vi "patientListView.vi"() -> ()   [LabVIEW 2019]
uses:
  03_Home/controller/logoutBtn.ctl
  03_Home/controller/exitBtn.ctl
  <vilib>/Utility/miscctls.llb/LVPointTypeDef.ctl
  subVI/patients_state.ctl
  03_Home/controller/pannelState.ctl
  globalValue.vi
panel:
  in  "btnGroup":T1
  in  "trashBtn":bool
  in  "createBtn":bool
  in  "backPage":bool
  out "x-y*floor(x/y)":i32
  out "totalCount":string
  out "totalPage":i8
  out "crrentPage":i8
  in  "leftBtn":bool
  in  "rightBtn":bool
  out "patientList":i32(listbox)
  in  "searchBtn":bool
  in  "searchForm":string
  in  "Help Button":bool
  in  "LogOut Button":T2
  in  "Exit Button":T3
  out "userNm":string
  # "/"
  # "|"
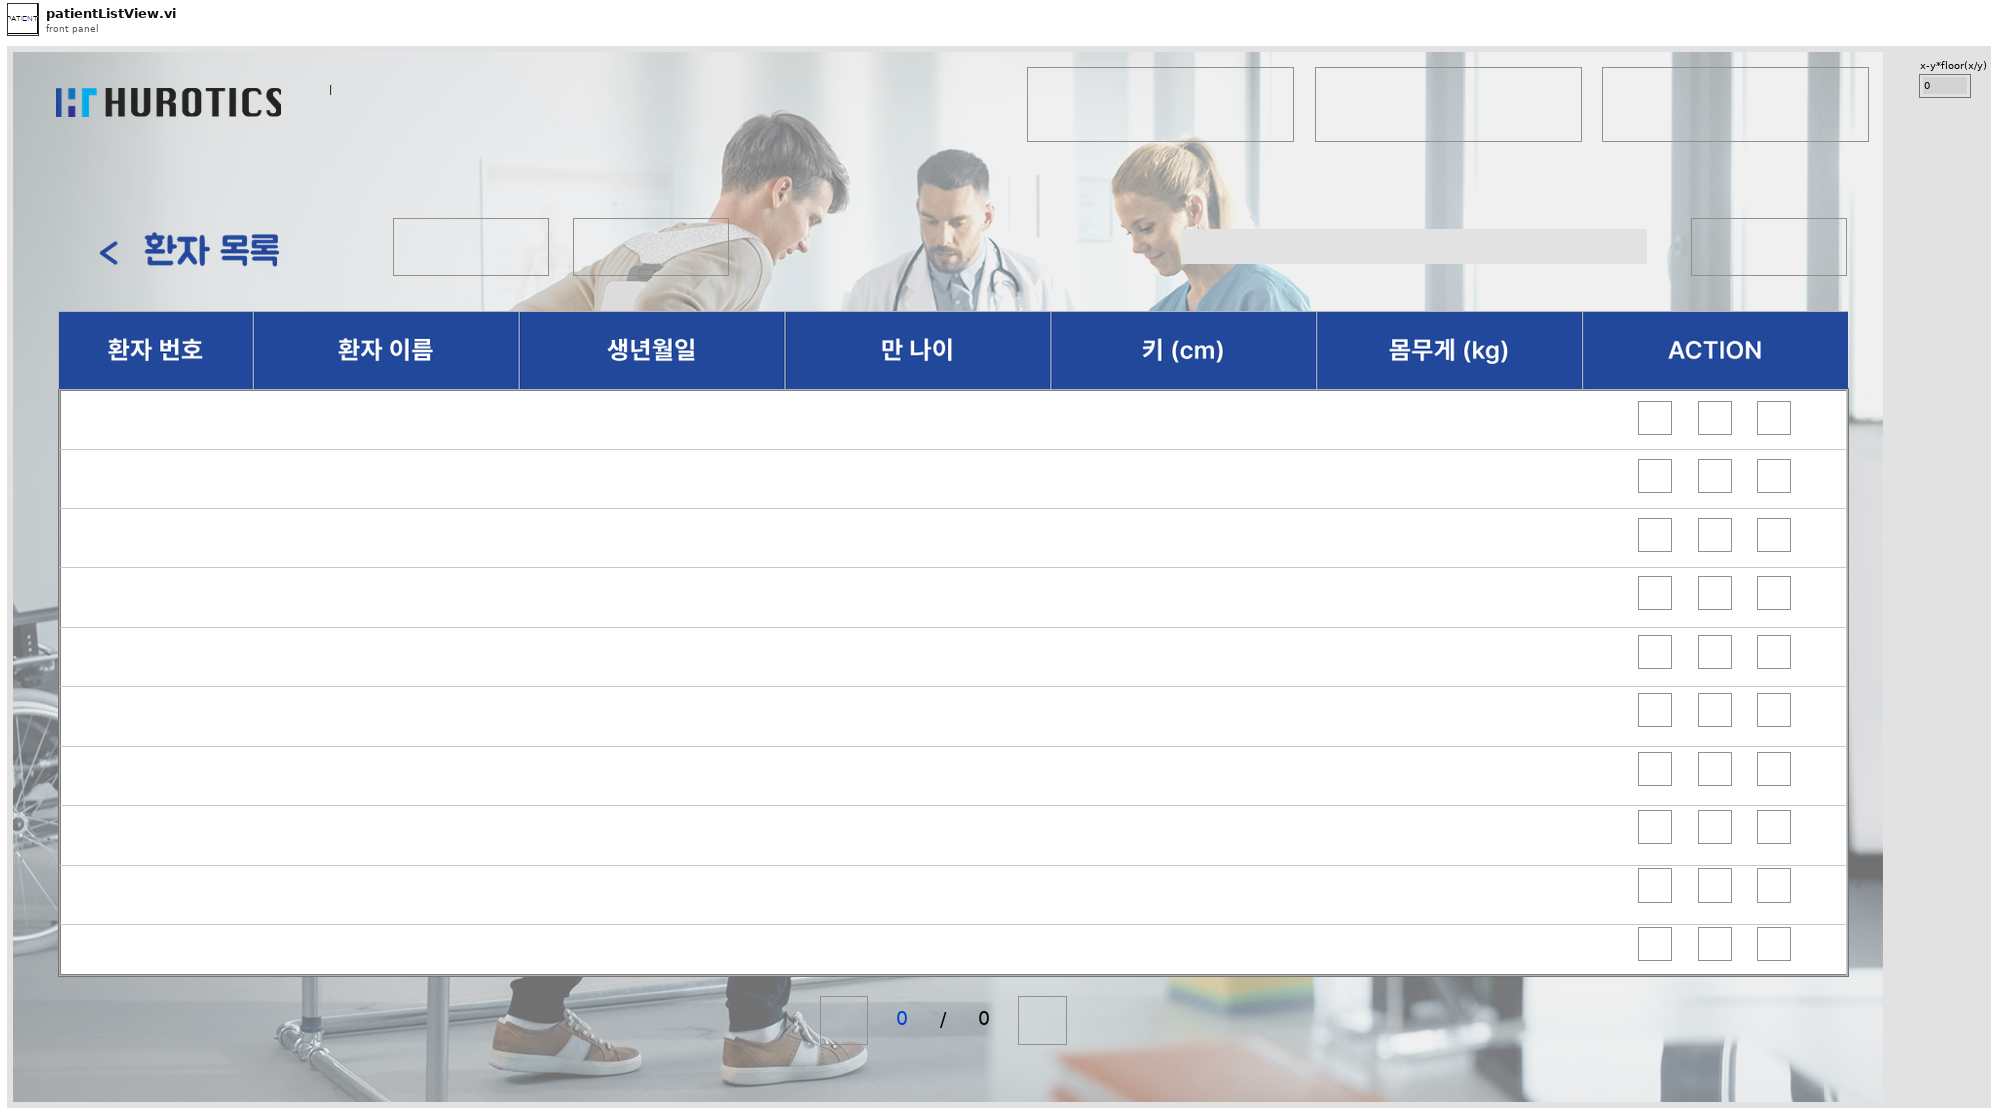
[diagram p1: front panel]
types:
  T1 = cluster{"detailBtn":bool, "updateBtn":bool, "deleteBtn":bool, "detailBtn 2":bool, "updateBtn 2":bool, "deleteBtn 2":bool, "detailBtn 3":bool, "updateBtn 3":bool, "deleteBtn 3":bool, "detailBtn 4":bool, "updateBtn 4":bool, "deleteBtn 4":bool, "detailBtn 5":bool, "updateBtn 5":bool, "deleteBtn 5":bool, "detailBtn 6":bool, "updateBtn 6":bool, "deleteBtn 6":bool, "detailBtn 7":bool, "updateBtn 7":bool, "deleteBtn 7":bool, "detailBtn 8":bool, "updateBtn 8":bool, "deleteBtn 8":bool, "detailBtn 9":bool, "updateBtn 9":bool, "deleteBtn 9":bool, "detailBtn 10":bool, "updateBtn 10":bool, "deleteBtn 10":bool}
  T2 = typedef "logoutBtn.ctl" = bool
  T3 = typedef "exitBtn.ctl" = bool
  T4 = typedef "LVPointTypeDef.ctl" = cluster{"Horizontal":i16, "Vertical":i16}
  T5 = enum16{"connection", "create", "getReadList", "getRead", "getCount", "update", "delete", "close"}
  T6 = typedef "patients_state.ctl" = enum16{"connection", "create", "getReadList", "getRead", "getCount", "update", "delete", "trash", "restore", "close"}
  T7 = enum8{"Enabled", "Disabled", "Disabled and Grayed Out"}
  T8 = typedef "pannelState.ctl" = enum16{"Init", "LogIn", "SignUpView", "Home", "Management_patientList", "Management_patientTrashtList", "Management_patientCreate", "Management_patientUpdate", "Management_patientTraining", "Management_patientTrainingDetail", "H-MEDI PatientList", "H-MEDI HardwareCtl", "Adjust", "FineTuning", "UserList", "UserDetail", "Exit"}
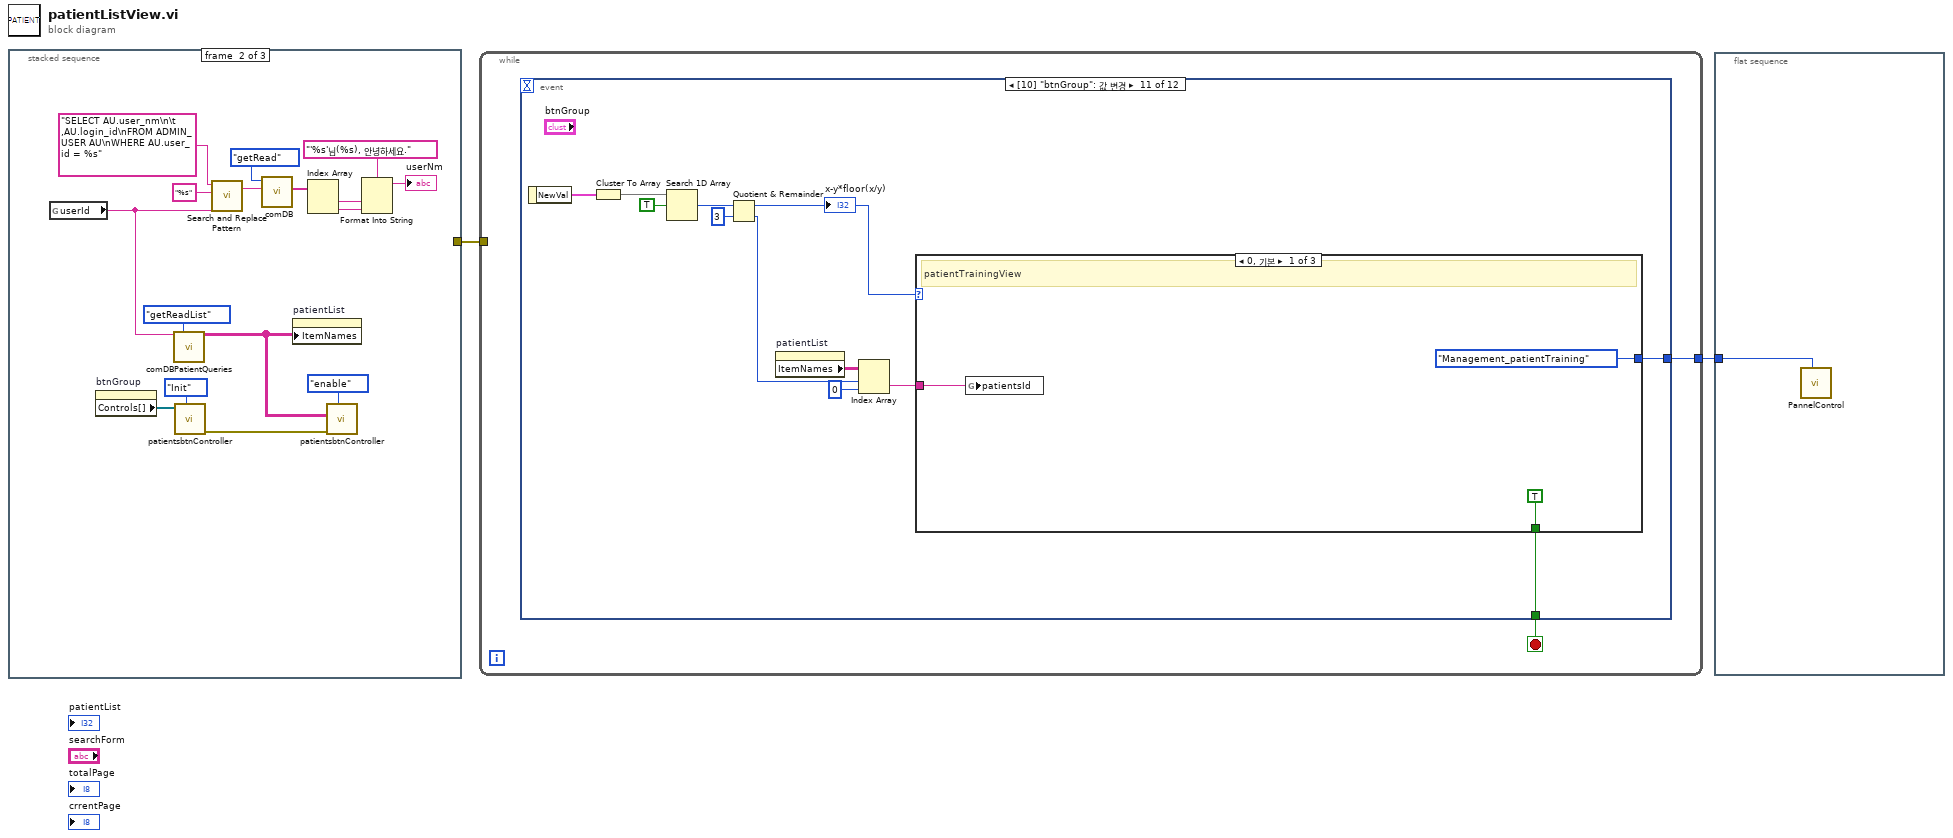
[diagram p0: block diagram]
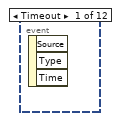
[diagram p2: hidden frame]
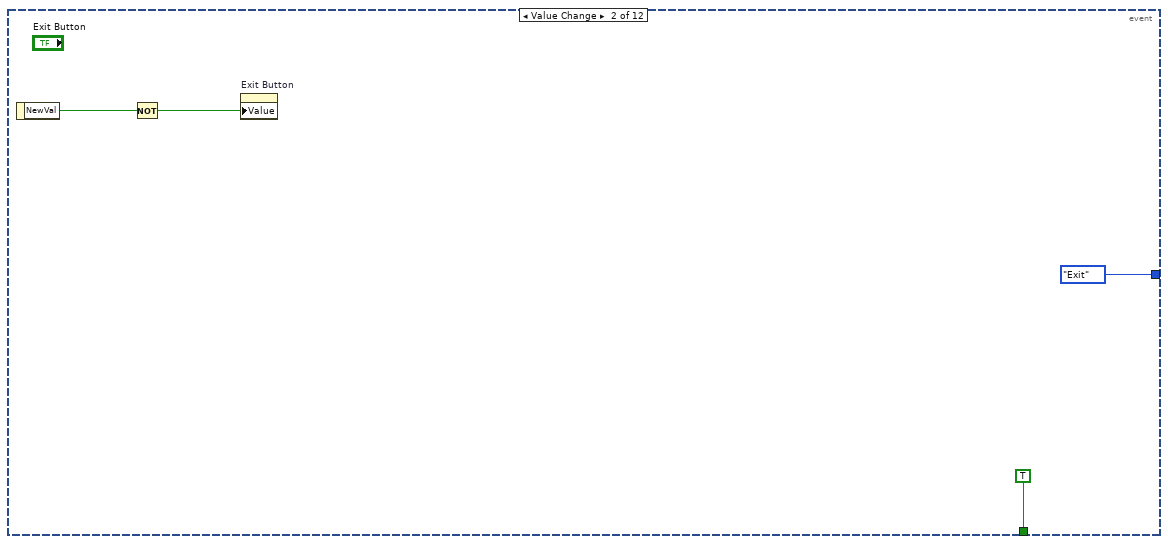
[diagram p3: hidden frame]
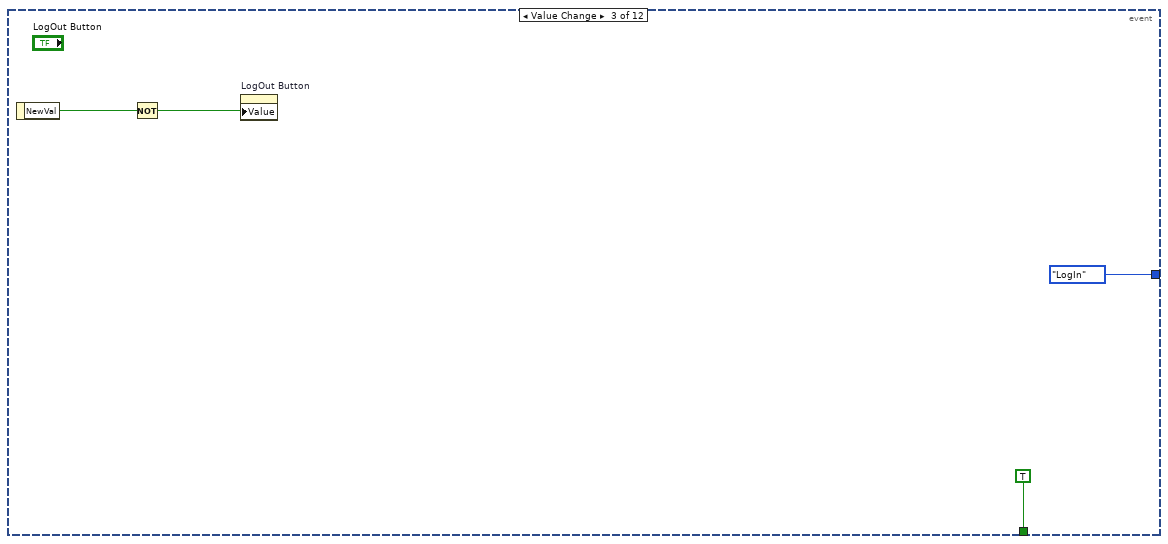
[diagram p4: hidden frame]
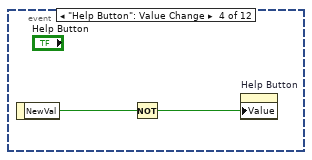
[diagram p5: hidden frame]
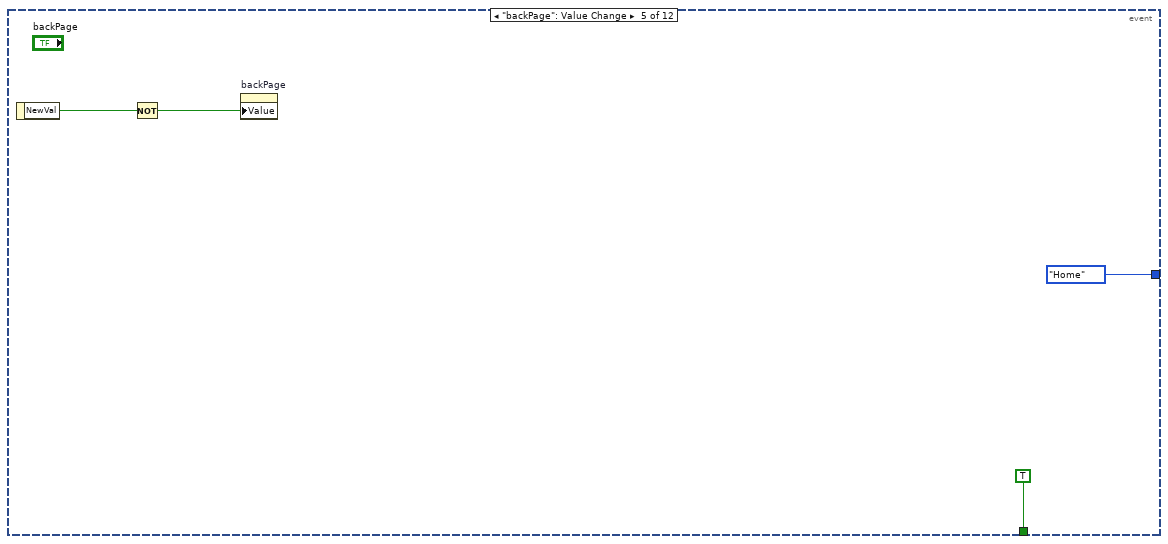
[diagram p6: hidden frame]
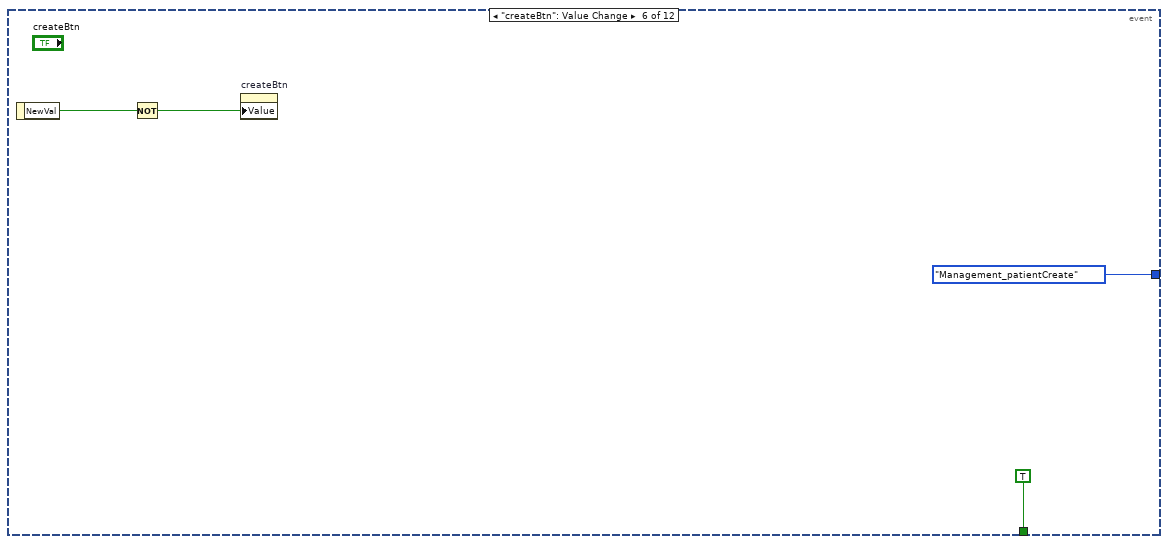
[diagram p7: hidden frame]
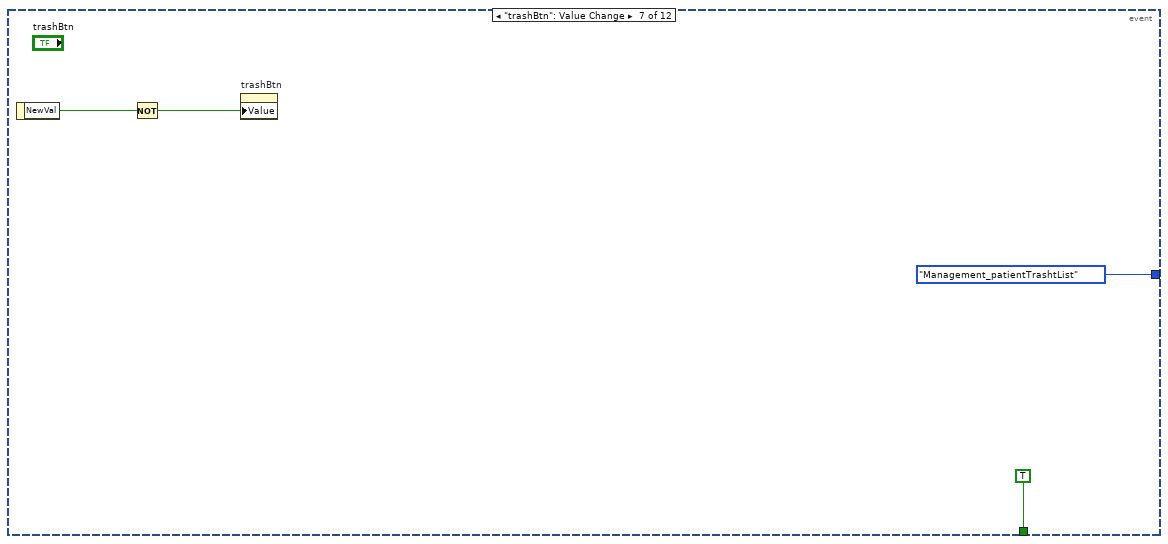
[diagram p8: hidden frame]
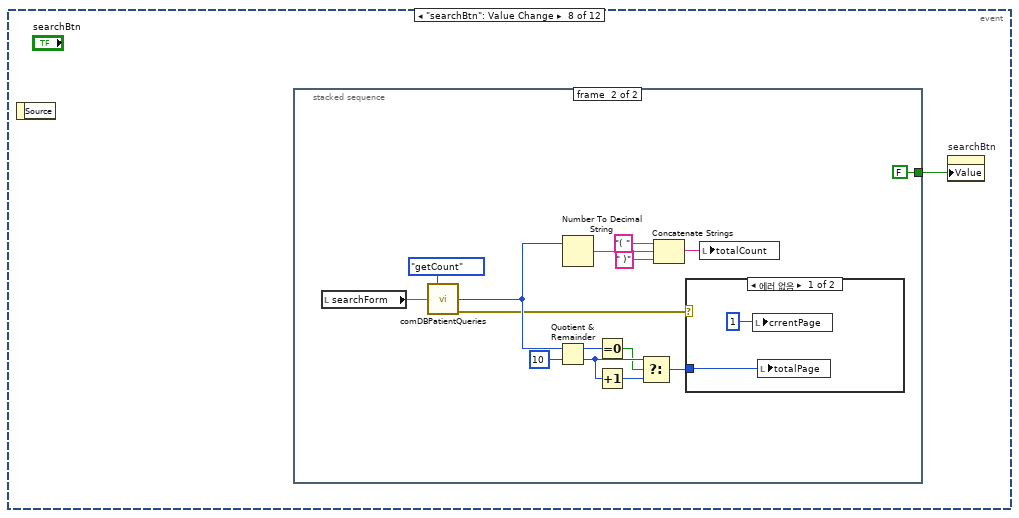
[diagram p9: hidden frame]
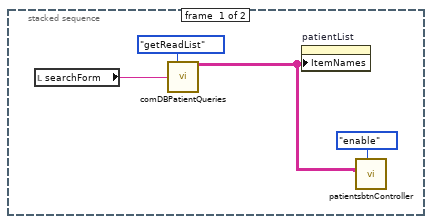
[diagram p10: hidden frame]
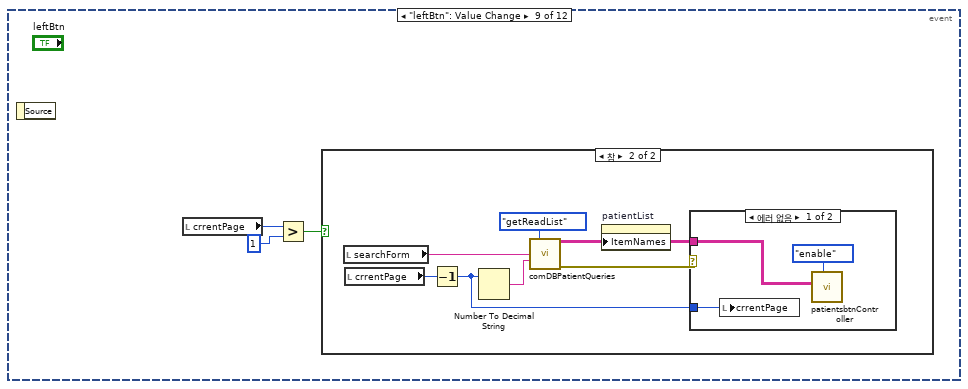
[diagram p12: hidden frame]
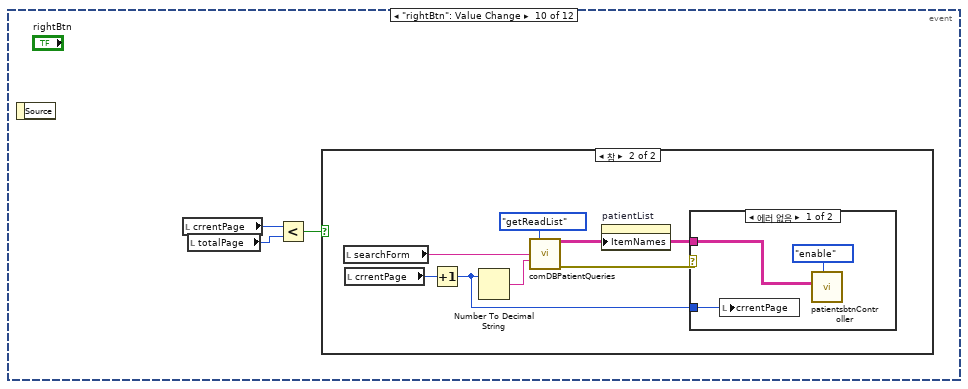
[diagram p15: hidden frame]
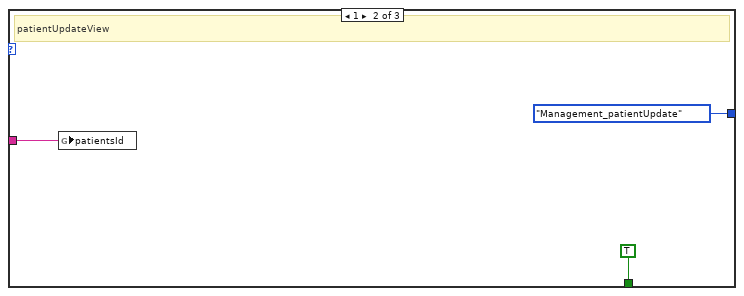
[diagram p18: hidden frame]
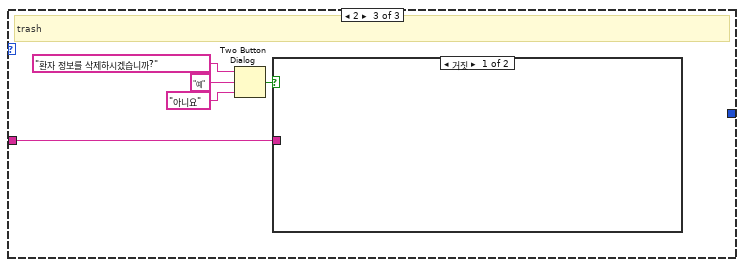
[diagram p19: hidden frame]
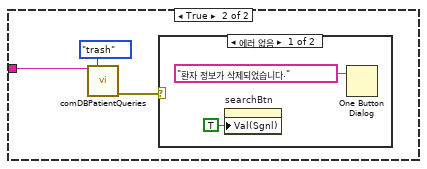
[diagram p20: hidden frame]
diagram:
  n1 = stacked-sequence {
    tunnel: [w6 _ _] -> w2
    frame #0 {
      w5 = T7."Disabled" ("비활성화")
      n2 = control-ref of="구획"() -> (w12:refnum<vi>)
      n3 = property class="Pane"(reference=w12, "Origin"=T4 {"Horizontal"=0, "Vertical"=0} ("원점")) -> (error out=w10:errorcluster)  [unwired: 1 in, 1 out]
      n4 = local write "patientList"(-1 ("userList")) -> ()
      n5 = local write "crrentPage"(i8 1 ("crrentPage")) -> ()
      n6 = local write "searchForm"("" ("searchForm")) -> ()
      n7 = local write "searchBtn"(FALSE ("searchBtn")) -> ()
      n8 = control-ref of="이 VI"() -> (w14:refnum<vi>)
      n9 = property class="VI"(reference=w14, error in=w10, "Front Panel.IsFrontmost"=TRUE ("프런트패널 윈도우:맨 앞으로")) -> (error out=w6:errorcluster)  [unwired: 1 out]
      n10 = property on="patientList" class="MCListbox (엄격한)"("ItemNames"=string[][] [] ("아이템 이름")) -> ()  [unwired: 2 in, 2 out]
      n11 = property on="userNm" class="Str"("DisabledEnum"=w5) -> ()  [unwired: 2 in, 2 out]
      n12 = property on="totalCount" class="Str"("DisabledEnum"=w5) -> ()  [unwired: 2 in, 2 out]
      n13 = property on="totalPage" class="DigNum (엄격한)"("DisabledEnum"=w5) -> ()  [unwired: 2 in, 2 out]
      n14 = property on="crrentPage" class="DigNum (엄격한)"("DisabledEnum"=w5) -> ()  [unwired: 2 in, 2 out]
    }
    frame #1 {
      n15 = global read "globalValue.vi" "userId"() -> (w15:string)
      n16 = property on="btnGroup" class="Clust"() -> ("Controls[]"=w27:refnum<vi>[])  [unwired: 2 in, 2 out]
      n17 = call "comDBPatientQueries.vi"("id"=w15, "State"=patients_state."getReadList") -> ("resultList"=w25:string[][])  [unwired: 10 in, 3 out]
      n18 = call "patientsbtnController.vi"("state"=enum16{"Init", "disable", "enable"}."Init", "Controls[]"=w27) -> ("error out"=w29:errorcluster)  [unwired: 9 in]
      n19 = call <vilib>:"Search and Replace Pattern.vi"("string"="SELECT AU.user_nm\n\t         ,AU.login_id\nFROM ADMIN_USER AU\nWHERE AU.user_id = %s" ("Query"), "regular expression (\"\")"="%s" ("regular expression (\"\")"), "replace string (\"\")"=w15) -> ("result string"=w17:string)  [unwired: 2 in, 1 out]
      n20 = call "comDB.vi"("Query"=w17, "State"=T5."getRead") -> ("result1DArray"=w22:string[])  [unwired: 5 in, 3 out]
      n21 = property on="patientList" class="MCListbox (엄격한)"("ItemNames"=w25) -> ()  [unwired: 2 in, 2 out]
      n22 = Index Array(array=w22) -> (element #1=w21:string, element #2=w20:string)  [unwired: 2 in]
      n23 = call "patientsbtnController.vi"("state"=enum16{"Init", "disable", "enable"}."enable", "error in (no error)"=w29, "2dArray"=w25) -> ()  [unwired: 8 in, 1 out]
      n24 = Format Into String(format string="'%s'님(%s), 안녕하세요." ("문자열"), w21, w20) -> (resulting string=→"userNm":string)  [unwired: 2 in, 1 out]
    }
    frame #2 {
      # "Total Page"
      n25 = call "comDBPatientQueries.vi"("State"=patients_state."getCount") -> ("count"=w31:i64)  [unwired: 11 in, 3 out]
      n26 = Quotient & Remainder(x=w31, y=i64 10) -> (x-y*floor(x/y)=w34:i64, floor(x/y)=w33:i64)
      n27 = Number To Decimal String(number=w31) -> (decimal integer string=w40:string)  [unwired: 1 in]
      n28 = Equal To 0?(x=w34) -> (x = 0?=w35:bool)
      n29 = Increment(x=w33) -> (x+1=w37:i64)
      n30 = Select(t=w33, s=w35, f=w37) -> (s? t:f=w36:i64)
      n31 = Concatenate Strings("( ", w40, " )") -> (→"totalCount":string)
      n32 = local write "totalPage"(w36) -> ()
    }
  }
  n33 = while {
    tunnel: w2 -> [_]
    tunnel: [w43] -> w1
    stop <- w44 stop-if-true
    n34 = event shown="[10] \"btnGroup\": 값 변경" {
      selector: _ -> [_ _ _ _ _ _ _ _ _ _ _ _]
      dyn-events: _ -> [_ _ _ _ _ _ _ _ _ _ _ _]
      timeout: _ -> [_ _ _ _ _ _ _ _ _ _ _ _]
      tunnel: [_ TRUE TRUE _ TRUE TRUE TRUE _ _ _ w119 w143] -> w44
      tunnel: [_ pannelState."Exit" ("State") pannelState."LogIn" ("State") _ pannelState."Home" ("State") pannelState."Management_patientCreate" ("State") pannelState."Management_patientTrashtList" ("State") _ _ _ w116 pannelState."Management_patientTraining" ("State")] -> w43
      event Timeout {
        n35 = event-data() -> ()  [unwired: 1 in, 3 out]
      }
      event Value Change {
        n36 = event-data() -> ("NewVal"=w46:T3)  [unwired: 1 in]
        n37 = Not(x=w46) -> (.not. x?=w45:T3)
        n38 = property on="Exit Button" class="Bool (엄격한)"("Value"=w45) -> ()  [unwired: 2 in, 2 out]
      }
      event Value Change {
        n39 = event-data() -> ("NewVal"=w52:T2)  [unwired: 1 in]
        n40 = Not(x=w52) -> (.not. x?=w51:T2)
        n41 = property on="LogOut Button" class="Bool (엄격한)"("Value"=w51) -> ()  [unwired: 2 in, 2 out]
      }
      event "Help Button": Value Change {
        n42 = event-data() -> ("NewVal"=w54:bool)  [unwired: 1 in]
        n43 = Not(x=w54) -> (.not. x?=w53:bool)
        n44 = property on="Help Button" class="Bool (엄격한)"("Value"=w53) -> ()  [unwired: 2 in, 2 out]
      }
      event "backPage": Value Change {
        n45 = event-data() -> ("NewVal"=w56:bool)  [unwired: 1 in]
        n46 = Not(x=w56) -> (.not. x?=w55:bool)
        n47 = property on="backPage" class="Bool (엄격한)"("Value"=w55) -> ()  [unwired: 2 in, 2 out]
      }
      event "createBtn": Value Change {
        n48 = event-data() -> ("NewVal"=w62:bool)  [unwired: 1 in]
        n49 = Not(x=w62) -> (.not. x?=w61:bool)
        n50 = property on="createBtn" class="Bool (엄격한)"("Value"=w61) -> ()  [unwired: 2 in, 2 out]
      }
      event "trashBtn": Value Change {
        n51 = event-data() -> ("NewVal"=w66:bool)  [unwired: 1 in]
        n52 = Not(x=w66) -> (.not. x?=w65:bool)
        n53 = property on="trashBtn" class="Bool (엄격한)"("Value"=w65) -> ()  [unwired: 2 in, 2 out]
      }
      event "searchBtn": Value Change {
        n54 = event-data() -> ()  [unwired: 1 in, 1 out]
        n55 = stacked-sequence {
          tunnel: [_ FALSE ("searchBtn")] -> w67
          frame #0 {
            n56 = local read "searchForm"() -> (w69:string)
            n57 = call "comDBPatientQueries.vi"("State"=patients_state."getReadList", "searchForm"=w69) -> ("resultList"=w68:string[][])  [unwired: 10 in, 3 out]
            n58 = property on="patientList" class="MCListbox (엄격한)"("ItemNames"=w68) -> ()  [unwired: 2 in, 2 out]
            n59 = call "patientsbtnController.vi"("state"=enum16{"Init", "disable", "enable"}."enable", "2dArray"=w68) -> ()  [unwired: 9 in, 1 out]
          }
          frame #1 {
            n60 = local read "searchForm"() -> (w74:string)
            n61 = call "comDBPatientQueries.vi"("State"=patients_state."getCount", "searchForm"=w74) -> ("count"=w73:i64, "error out"=w72:errorcluster)  [unwired: 10 in, 2 out]
            n62 = Quotient & Remainder(x=w73, y=i64 10) -> (x-y*floor(x/y)=w78:i64, floor(x/y)=w79:i64)
            n63 = Number To Decimal String(number=w73) -> (decimal integer string=w83:string)  [unwired: 1 in]
            n64 = Equal To 0?(x=w78) -> (x = 0?=w77:bool)
            n65 = Increment(x=w79) -> (x+1=w81:i64)
            n66 = Select(t=w79, s=w77, f=w81) -> (s? t:f=w80:i64)
            n67 = Concatenate Strings("( ", w83, " )") -> (w84:string)
            n68 = case shown="에러 없음" w72 {
              tunnel: w80 -> [w87 _]
              frame No Error {
                n69 = local write "crrentPage"(i8 1 ("crrentPage")) -> ()
                n70 = local write "totalPage"(w87) -> ()
              }
              frame Error {
              }
            }
            n71 = local write "totalCount"(w84) -> ()
          }
        }
        n72 = property on="searchBtn" class="Bool (엄격한)"("Value"=w67) -> ()  [unwired: 2 in, 2 out]
      }
      event "leftBtn": Value Change {
        n73 = event-data() -> ()  [unwired: 1 in, 1 out]
        n74 = local read "crrentPage"() -> (w89:i8)
        n75 = Greater?(x=w89, y=1) -> (0:w91:bool)
        n76 = case shown="참" w91 {
          frame False {
          }
          frame True {
            n77 = local read "searchForm"() -> (w95:string)
            n78 = local read "crrentPage"() -> (w98:i8)
            n79 = Decrement(x=w98) -> (x-1=w97:i8)
            n80 = Number To Decimal String(number=w97) -> (decimal integer string=w94:string)  [unwired: 1 in]
            n81 = call "comDBPatientQueries.vi"("State"=patients_state."getReadList", "searchForm"=w95, "crrentPage"=w94) -> ("resultList"=w92:string[][], "error out"=w93:errorcluster)  [unwired: 9 in, 2 out]
            n82 = property on="patientList" class="MCListbox (엄격한)"("ItemNames"=w92) -> ()  [unwired: 2 in, 2 out]
            n83 = case shown="에러 없음" w93 {
              tunnel: w97 -> [w101 _]
              tunnel: w92 -> [w99 _]
              frame No Error {
                n84 = local write "crrentPage"(w101) -> ()
                n85 = call "patientsbtnController.vi"("state"=enum16{"Init", "disable", "enable"}."enable", "2dArray"=w99) -> ()  [unwired: 9 in, 1 out]
              }
              frame Error {
              }
            }
          }
        }
      }
      event "rightBtn": Value Change {
        n86 = event-data() -> ()  [unwired: 1 in, 1 out]
        n87 = local read "crrentPage"() -> (w104:i8)
        n88 = local read "totalPage"() -> (w103:i8)
        n89 = Less?(x=w104, y=w103) -> (x < y?=w102:bool)
        n90 = case shown="참" w102 {
          frame False {
          }
          frame True {
            n91 = local read "searchForm"() -> (w108:string)
            n92 = local read "crrentPage"() -> (w111:i8)
            n93 = Increment(x=w111) -> (x+1=w110:i8)
            n94 = Number To Decimal String(number=w110) -> (decimal integer string=w107:string)  [unwired: 1 in]
            n95 = call "comDBPatientQueries.vi"("State"=patients_state."getReadList", "searchForm"=w108, "crrentPage"=w107) -> ("resultList"=w105:string[][], "error out"=w106:errorcluster)  [unwired: 9 in, 2 out]
            n96 = property on="patientList" class="MCListbox (엄격한)"("ItemNames"=w105) -> ()  [unwired: 2 in, 2 out]
            n97 = case shown="에러 없음" w106 {
              tunnel: w110 -> [w114 _]
              tunnel: w105 -> [w112 _]
              frame No Error {
                n98 = local write "crrentPage"(w114) -> ()
                n99 = call "patientsbtnController.vi"("state"=enum16{"Init", "disable", "enable"}."enable", "2dArray"=w112) -> ()  [unwired: 9 in, 1 out]
              }
              frame Error {
              }
            }
          }
        }
      }
      event "btnGroup": Value Change {
        n100 = event-data() -> ("NewVal"=w118:T1)  [unwired: 1 in]
        n101 = Cluster To Array(cluster=w118) -> (array=w126:bool[])
        n102 = Search 1D Array(1D array=w126, element=TRUE ("원소")) -> (index of element=w125:i32)  [unwired: 1 in]
        n103 = Quotient & Remainder(x=w125, y=3) -> (x-y*floor(x/y)=w120:i32, floor(x/y)=w121:i32)
        "x-y*floor(x/y)" <- w120
        n104 = property on="patientList" class="MCListbox (엄격한)"() -> ("ItemNames"=w123:string[][])  [unwired: 2 in, 2 out]
        n105 = Index Array(array=w123, index (row)=w121, index (col)=0 ("비활성화된 인덱스 (열)")) -> (element=w115:string)
        n106 = case shown="0, 기본" w120 {
          tunnel: w115 -> [w127 w130 w134]
          tunnel: [TRUE TRUE _] -> w119
          tunnel: [pannelState."Management_patientTraining" ("State") pannelState."Management_patientUpdate" ("State") _] -> w116
          frame 0, Default {
            # "patientTrainingView"
            n107 = global write "globalValue.vi" "patientsId"(w127) -> ()
          }
          frame 1 {
            # "patientUpdateView"
            n108 = global write "globalValue.vi" "patientsId"(w130) -> ()
          }
          frame 2 {
            # "trash"
            n109 = Two Button Dialog(message="환자 정보를 삭제하시겠습니까?" ("메시지"), 1:"아니요" ("거짓 버튼 이름(\"취소\")"), 2:"예" ("참 버튼 이름(\"확인\")")) -> (T button?=w133:bool)
            n110 = case shown="거짓" w133 {
              tunnel: w134 -> [_ w139]
              frame False {
              }
              frame True {
                n111 = call "comDBPatientQueries.vi"("id"=w139, "State"=patients_state."trash") -> ("error out"=w138:errorcluster)  [unwired: 10 in, 3 out]
                n112 = case shown="에러 없음" w138 {
                  frame No Error {
                    n113 = property on="searchBtn" class="Bool (엄격한)"("Val(Sgnl)"=TRUE ("값(신호)")) -> ()  [unwired: 2 in, 2 out]
                    n114 = One Button Dialog(message="환자 정보가 삭제되었습니다." ("메시지")) -> ()  [unwired: 1 in, 1 out]
                  }
                  frame Error {
                  }
                }
              }
            }
          }
        }
      }
      event "patientList": Double Click {
        n115 = event-data() -> ("Row"=w146:i32)  [unwired: 1 in]
        n116 = property on="patientList" class="MCListbox (엄격한)"() -> ("ItemNames"=w148:string[][])  [unwired: 2 in, 2 out]
        n117 = Index Array(array=w148, index (row)=w146, index (col)=0 ("비활성화된 인덱스 (열)")) -> (element=w145:string)
        n118 = Empty String/Path?(string/path=w145) -> (empty?=w144:bool)
        n119 = case shown="거짓" w144 {
          tunnel: w145 -> [w151 _]
          tunnel: [TRUE _] -> w143
          frame False {
            n120 = global write "globalValue.vi" "patientsId"(w151) -> ()
          }
          frame True {
          }
        }
      }
    }
  }
  n121 = flat-sequence {
    tunnel: w1 -> [w152]
    frame #0 {
      n122 = call "PannelControl.vi"("State"=w152) -> ()  [unwired: 10 in, 1 out]
    }
  }
